vi "ep_Replace Range Utilization (Single Line).vi"(8 "error in (no error)":errorcluster, 9 "system info in":refnum<class "EP System Info.lvclass">, 10 "full-range RMS values":dbl[](array[numeric]), 11 "waveforms in":waveform(dbl)[](array[waveform])) -> (0 "error out":errorcluster, 1 "system info out":refnum<class "EP System Info.lvclass">, 3 "actual ranges [%]":dbl[](array[numeric]))   [LabVIEW 2014, in "NI_EP_Power Quality.lvlib"]
uses:
  <vilib>/addons/Electrical Power/PQ/NI_EP_Power Quality.lvlib
  <vilib>/addons/Electrical Power/PQ/Common/Classes/System Info/EP System Info.lvclass
  <vilib>/addons/Electrical Power/PQ/Common/Controls/ep_AI Data Channel.ctl
  <vilib>/Analysis/5stat.llb/RMS (DBL).vi
  <vilib>/Analysis/NI_AALPro.lvlib
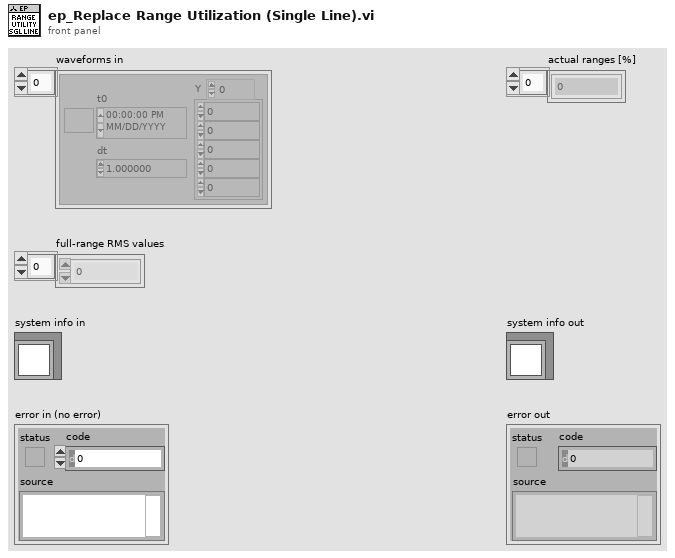
[diagram p1: front panel]
types:
  T1 = typedef "NI_EP_Power Quality.lvlib/ep_AI Data Channel.ctl" = enum16{"Voltage Phase A (L1)", "Voltage Phase B (L2)", "Voltage Phase C (L3)", "Voltage Phase N (Neutral)", "Current Phase A (L1)", "Current Phase B (L2)", "Current Phase C (L3)", "Current Phase N (Neutral)"}
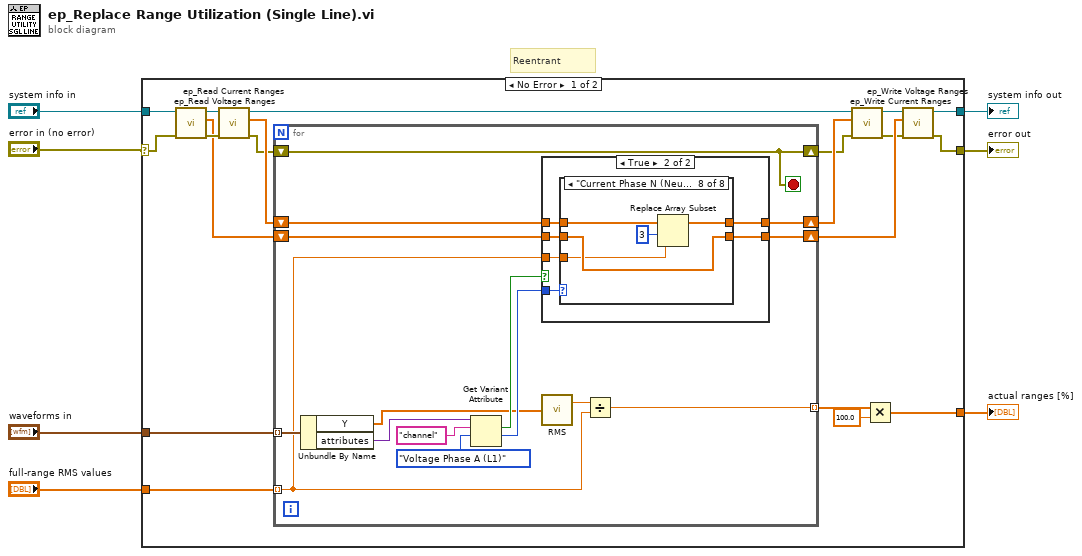
[diagram p0: block diagram]
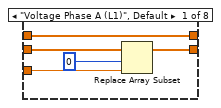
[diagram p3: hidden frame]
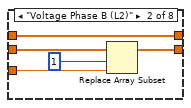
[diagram p4: hidden frame]
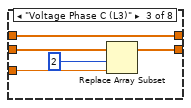
[diagram p5: hidden frame]
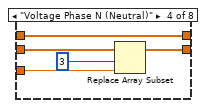
[diagram p6: hidden frame]
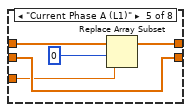
[diagram p7: hidden frame]
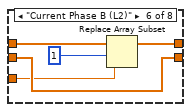
[diagram p8: hidden frame]
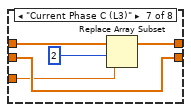
[diagram p9: hidden frame]
diagram:
  # "Reentrant"
  n1 = case shown="No Error" "error in (no error)" {
    selector: "error in (no error)" -> [w10 w92]
    tunnel: "system info in" -> [w16 w91]
    tunnel: "waveforms in" -> [w15 _]
    tunnel: "full-range RMS values" -> [w14 _]
    tunnel: [w13 _] -> w4
    tunnel: [w12 w91] -> w3
    tunnel: [w11 w92] -> w2
    frame No Error {
      n2 = call <vilib>:"ep_Read Voltage Ranges.vi"("error in (no error)"=w10, "system info in"=w16) -> ("error out"=w26:errorcluster, "voltage ranges"=w19:dbl[], "system info out"=w27:refnum<class "EP System Info.lvclass">)  [unwired: 7 in]
      n3 = call <vilib>:"ep_Read Current Ranges.vi"("error in (no error)"=w26, "system info in"=w27) -> ("error out"=w9:errorcluster, "current ranges"=w25:dbl[], "system info out"=w21:refnum<class "EP System Info.lvclass">)  [unwired: 7 in]
      n4 = for {
        tunnel: w15 -> [w42] mode=indexing
        tunnel: [w37] -> w17 mode=indexing
        shift-right: [w34] -> w23
        shift-left: w19 -> [w35]
        shift-right: [w33] -> w24
        shift-left: w25 -> [w32]
        tunnel: w14 -> [w36] mode=indexing
        shift-right: [w28] -> w8
        shift-left: w9 -> [w28]
        stop <- w28 stop-if-true
        n5 = Unbundle By Name(w42) -> ("Y"=w29:dbl[], "attributes"=w30:variant)
        n6 = Get Variant Attribute(Variant=w30, name="channel", default value (empty Variant)=ep_AI_Data_Channel."Voltage Phase A (L1)" ("AI data channel")) -> (found=w40:bool, value=w39:T1)  [unwired: 1 in, 2 out]
        n7 = case shown="True" w40 {
          tunnel: w39 -> [_ w50]
          tunnel: w36 -> [_ w49]
          tunnel: w35 -> [w44 w48]
          tunnel: [w44 w45] -> w34
          tunnel: [w43 w47] -> w33
          tunnel: w32 -> [w43 w46]
          frame False {
          }
          frame True {
            n8 = case shown="\"Current Phase N (Neutral)\"" w50 {
              tunnel: w49 -> [w54 w59 w64 w69 w71 w76 w81 w86]
              tunnel: w48 -> [w55 w60 w65 w70 w72 w77 w82 w87]
              tunnel: [w53 w58 w63 w68 w73 w78 w83 w88] -> w47
              tunnel: w46 -> [w53 w58 w63 w68 w74 w79 w84 w89]
              tunnel: [w52 w57 w62 w67 w72 w77 w82 w87] -> w45
              frame "Voltage Phase A (L1)", Default {
                n9 = Replace Array Subset(array=w55, new element=w54, index=0) -> (w52:dbl[])
              }
              frame "Voltage Phase B (L2)" {
                n10 = Replace Array Subset(array=w60, new element=w59, index=1) -> (w57:dbl[])
              }
              frame "Voltage Phase C (L3)" {
                n11 = Replace Array Subset(array=w65, new element=w64, index=2) -> (w62:dbl[])
              }
              frame "Voltage Phase N (Neutral)" {
                n12 = Replace Array Subset(array=w70, new element=w69, index=3) -> (w67:dbl[])
              }
              frame "Current Phase A (L1)" {
                n13 = Replace Array Subset(array=w74, new element=w71, index=0) -> (w73:dbl[])
              }
              frame "Current Phase B (L2)" {
                n14 = Replace Array Subset(array=w79, new element=w76, index=1) -> (w78:dbl[])
              }
              frame "Current Phase C (L3)" {
                n15 = Replace Array Subset(array=w84, new element=w81, index=2) -> (w83:dbl[])
              }
              frame "Current Phase N (Neutral)" {
                n16 = Replace Array Subset(array=w89, new element=w86, index=3) -> (w88:dbl[])
              }
            }
          }
        }
        n17 = call-poly <vilib>:"RMS.vi"("X"=w29) -> ("rms value"=w38:dbl)  [unwired: 1 out]
        n18 = Divide(x=w38, y=w36) -> (x/y=w37:dbl)
      }
      n19 = call <vilib>:"ep_Write Current Ranges.vi"("error in (no error)"=w8, "current ranges"=w24, "system info in"=w21) -> ("error out"=w20:errorcluster, "system info out"=w22:refnum<class "EP System Info.lvclass">)  [unwired: 7 in]
      n20 = Multiply(x=w17, y=100.0) -> (x*y=w13:dbl[])
      n21 = call <vilib>:"ep_Write Voltage Ranges.vi"("error in (no error)"=w20, "voltage ranges"=w23, "system info in"=w22) -> ("error out"=w11:errorcluster, "system info out"=w12:refnum<class "EP System Info.lvclass">)  [unwired: 7 in]
    }
    frame Error {
    }
  }
  "error out" <- w2
  "actual ranges [%]" <- w4
  "system info out" <- w3
